vi "VMP_TestStand.vi"() -> ()   [LabVIEW 2016]
uses:
  <vilib>/userdefined/High Color/IMAQdx.ctl
  Enum_TypeDefinitions/Enum_TypeDef_FidMarkers.ctl
  Enum_TypeDefinitions/Enum_TypeDef_Sensors.ctl
  <vilib>/vision/Image Controls.llb/IMAQ Image.ctl
  <vilib>/Utility/file.llb/Read Delimited Spreadsheet (DBL).vi
  <vilib>/vision/driver/NI_Vision_Acquisition_Software.lvlib
panel:
  out "Module Progress Report":T1(array[cluster])
  in  "Reports path":path=path "C:/Users/Aerotech/cernbox/BNL/Stave Assembly Records/2017-05-10/ModulePlacement/5-11-2017"
  in  "Tab Control":enum32{"Camera", "Error handling"}(tab)
  in  "Camera Name":T2="cam1" caption="IMAQdx Session"
  in  "Camera gain":dbl
  in  "Module fiducial marker":T3
  in  "N modules":i32=2
  in  "Sensor Pattern":T4=enum."ATLAS12"
  out "Camera error out":errorcluster
  out "error out":errorcluster
  in  "Coordinates file path (dialog if empty)":path
  in  "Current module #":string
  in  "Current build phase":string
  in  "Axis Speeds":T5={"X [mm/s]"=25.0, "Y [mm/s]"=12.5, "Z [mm/s]"=5.0}
  in  "terminate":bool
  out "Current field of view":T6(plugin-control)
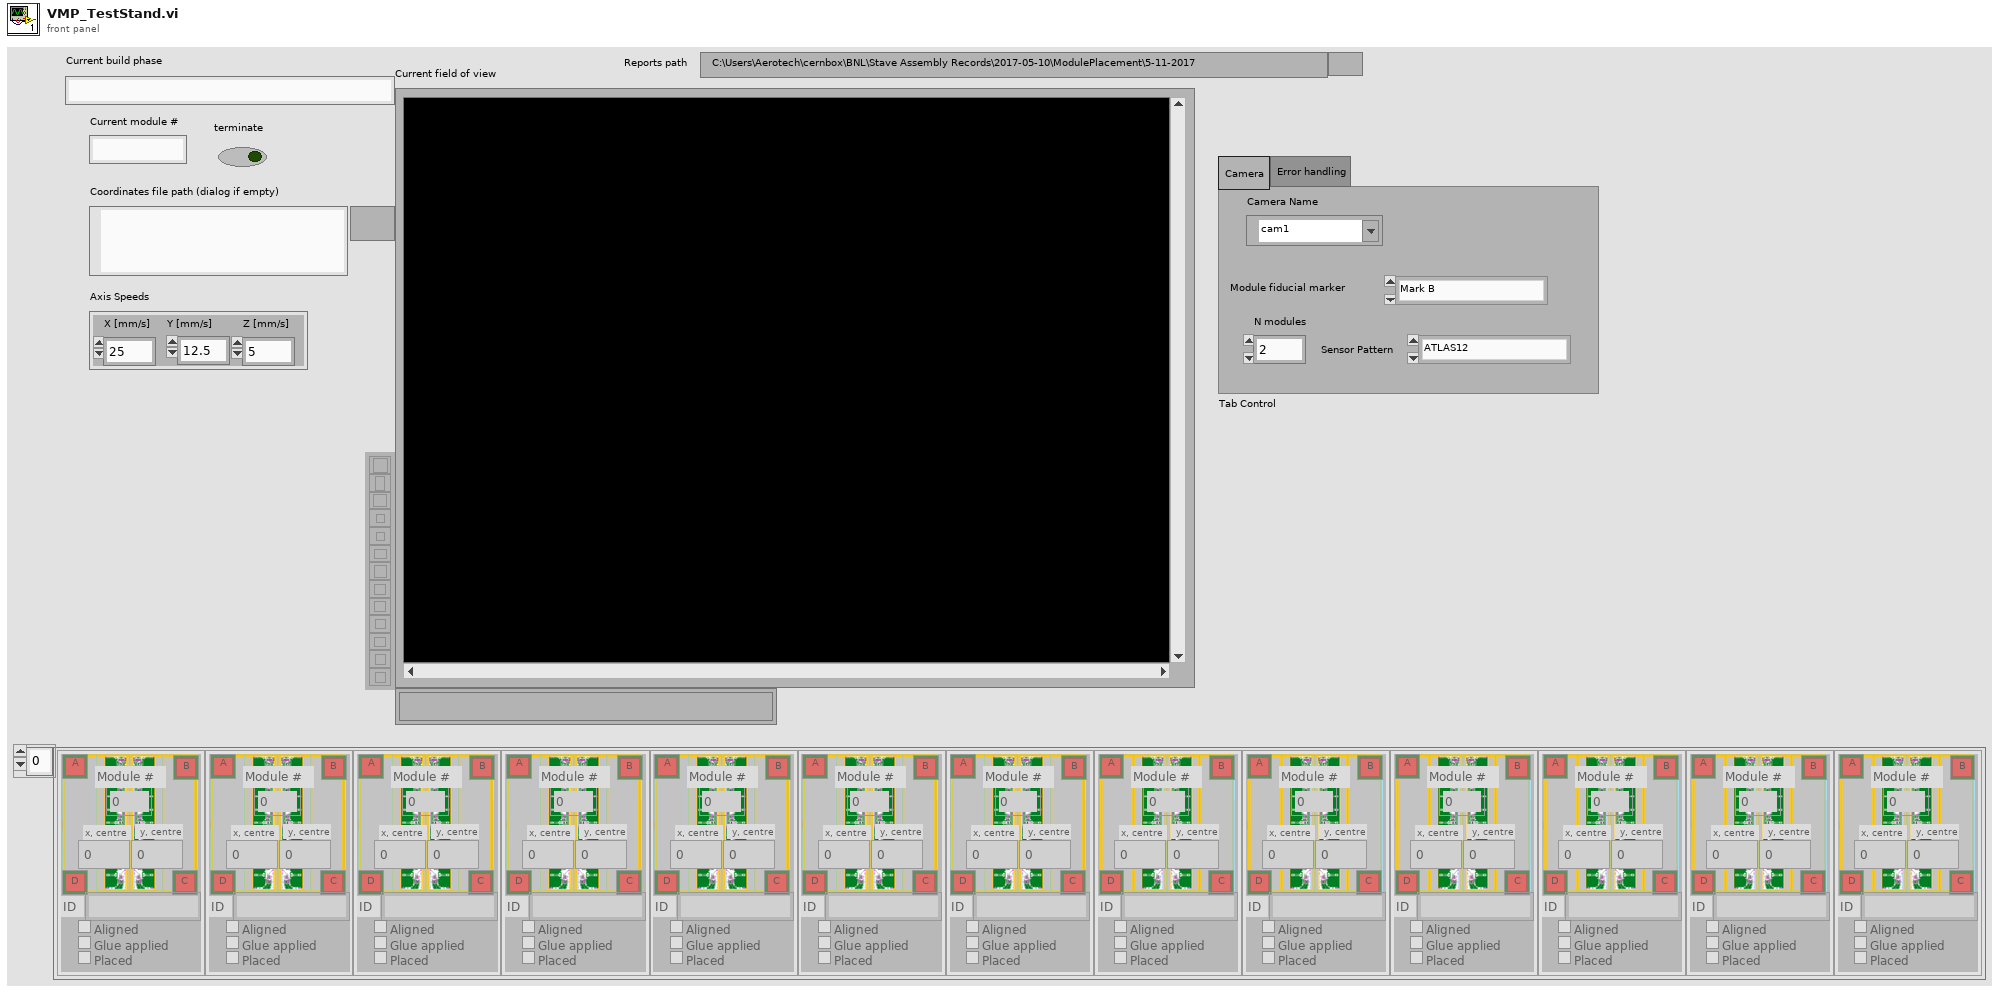
[diagram p1: front panel]
types:
  T1 = cluster{"B":bool, "A":bool, "D":bool, "C":bool, "ID":string, "Module #":i32, "x, centre":dbl, "y, centre":dbl, "Aligned":bool, "Glue applied":bool, "Placed":bool}[]
  T2 = typedef "IMAQdx.ctl" = refnum<k21>
  T3 = typedef "Enum_TypeDef_FidMarkers.ctl" = enum16{"Mark B", "Mark C", "Strip Corner", "Mark I (Slim/17)", "Mark E (Slim/17)", "Mark F (Slim/17)", "Mark G (Slim/17)", "Mark A (12)", "KaptonSpacers"}
  T4 = typedef "Enum_TypeDef_Sensors.ctl" = enum16{"ATLAS07", "ATLAS12", "ATLAS12Slim", "ATLAS17LS"}
  T5 = cluster{"X [mm/s]":dbl, "Y [mm/s]":dbl, "Z [mm/s]":dbl}
  T6 = typedef "IMAQ Image.ctl" = refnum<image>
  T7 = typedef "Image Type" = u32
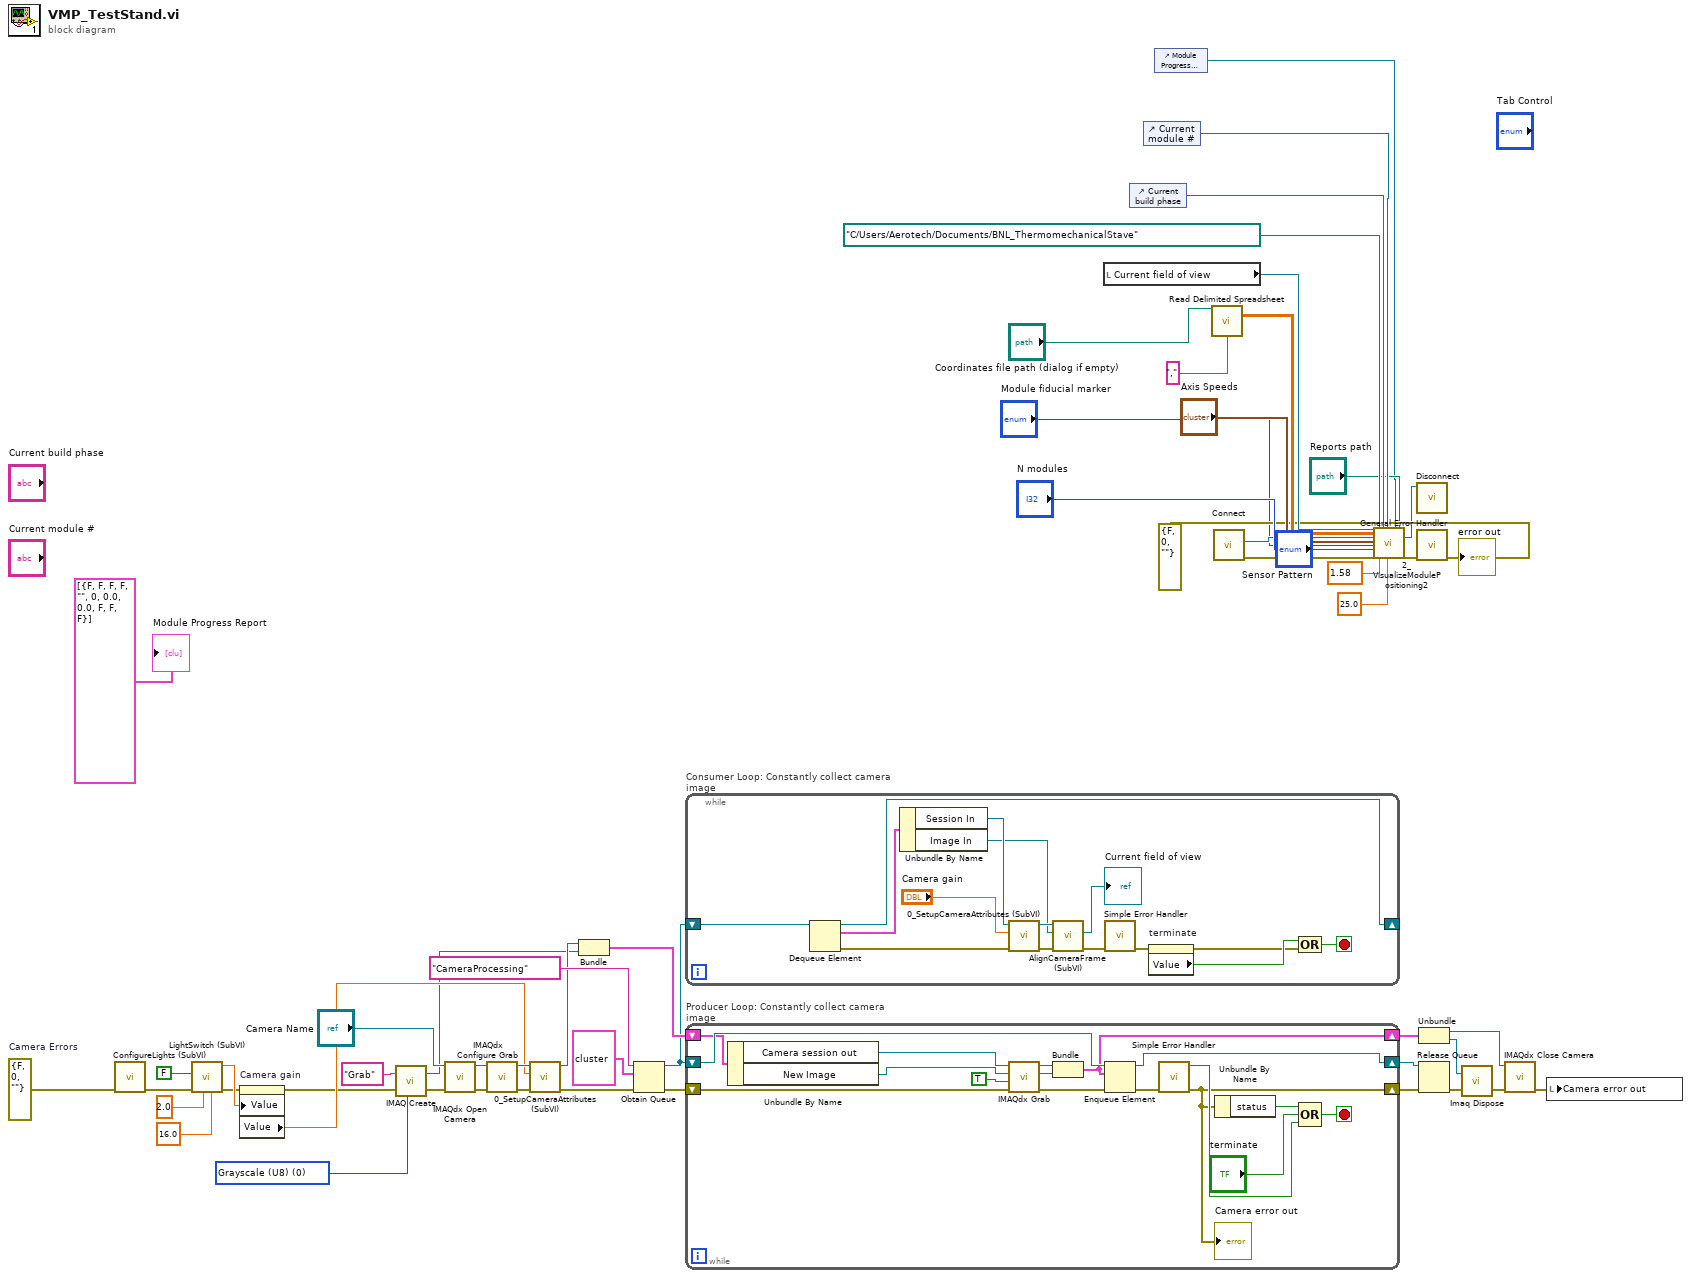
[diagram p0: block diagram]
diagram:
  w25 = errorcluster {"status"=FALSE, "code"=0, "source"=""}  # Camera Errors
  w53 = T7 0 items=["Grayscale (U8)", "Grayscale (I16)", "Grayscale (SGL)", "Complex (CSG)", "RGB (U32)", "HSL (U32)", "RGB (U64)", "Grayscale (U16)"] ("Image Type")
  n1 = call "ConfigureLights (SubVI).vi"("error in"=w25) -> ("error out"=w24:errorcluster)  [unwired: 10 in]
  n2 = call "LightSwitch (SubVI).vi"("Stave Gain"=16.0, "Si Gain"=2.0, "error in"=w24, "Spotlight"=FALSE) -> ("error out"=w45:errorcluster, "Assigned camera gain"=w46:dbl)  [unwired: 5 in, 1 out]
  n3 = property on="Camera gain" class="DigNum (strict)"(error in=w45, "Value"=w46) -> (error out=w23:errorcluster, "Value"=w40:dbl)  [unwired: 1 in, 1 out]
  n4 = call "IMAQ Create"("Image Name"="Grab", "Image Type"=w53, "error in (no error)"=w23) -> ("New Image"=w36:T6, "error out"=w50:errorcluster)  [unwired: 1 in, 1 out]
  n5 = call <vilib>:"IMAQdx Open Camera.vi"("error in"=w50, "Session In"="Camera Name") -> ("error out"=w51:errorcluster, "Session Out"=w54:T2)  [unwired: 1 in, 7 out]
  n6 = call <vilib>:"IMAQdx Configure Grab.vi"("error in"=w51, "Session In"=w54) -> ("error out"=w41:errorcluster, "Session Out"=w42:T2)  [unwired: 8 out]
  n7 = call "0_SetupCameraAttributes (SubVI).vi"("error in (no error)"=w41, "Gain"=w40, "Camera session in"=w42) -> ("error out"=w39:errorcluster, "Camera session out"=w37:T2)  [unwired: 7 in]
  n8 = Bundle("Camera session out"=w37, "New Image"=w36) -> (w35:cluster{"Camera session out":T2, "New Image":T6})  [unwired: 1 in]
  n9 = Obtain Queue(name (unnamed)="CameraProcessing", element data type=cluster{"Session In":T2, "Image In":T6} {"Session In"="", "Image In"=refnum}, error in (no error)=w39) -> (queue out=w27:refnum<queue>, error out=w38:errorcluster)  [unwired: 2 in, 1 out]
  n10 = while "Consumer Loop: Constantly collect camera image" {
    shift-right: [w65] -> _
    shift-left: w27 -> [w70]
    stop <- w68 stop-if-true
    n11 = Dequeue Element(queue=w70) -> (queue out=w65:refnum<queue>, element=w69:cluster{"Session In":T2, "Image In":T6}, error out=w67:errorcluster)  [unwired: 2 in, 1 out]
    n12 = Unbundle By Name(w69) -> ("Session In"=w64:T2, "Image In"=w62:T6)
    n13 = call "0_SetupCameraAttributes (SubVI).vi"("error in (no error)"=w67, "Gain"="Camera gain", "Camera session in"=w64) -> ("error out"=w61:errorcluster, "Camera session out"=w63:T2)  [unwired: 7 in]
    n14 = call "AlignCameraFrame (SubVI).vi"("error in (no error)"=w61, "Image Src"=w62, "Camera session in"=w63) -> ("error out"=w59:errorcluster, "Image Dst Out"=→"Current field of view":T6)  [unwired: 6 in, 1 out]
    n15 = call <vilib>:"Simple Error Handler.vi"("error in (no error)"=w59) -> ("error out"=w58:errorcluster)  [unwired: 4 in, 4 out]
    n16 = property on="terminate" class="Bool (strict)"(error in=w58) -> (error out=w57:errorcluster, "Value"=w66:bool)  [unwired: 1 in, 1 out]
    n17 = Compound Arithmetic op=OR(w66, w57) -> (w68:bool)
  }
  n18 = while "Producer Loop: Constantly collect camera image" {
    shift-right: [w84] -> w34
    shift-left: w27 -> [w85]
    shift-right: [w73] -> w33
    shift-left: w38 -> [w86]
    shift-right: [w75] -> w32
    shift-left: w35 -> [w78]
    stop <- w74 stop-if-true
    n19 = Unbundle By Name(w78) -> ("Camera session out"=w77:T2, "New Image"=w76:T6)
    n20 = call <vilib>:"IMAQdx Grab.vi"("error in"=w86, "Wait for Next Buffer? (Yes)"=TRUE, "Image In"=w76, "Session In"=w77) -> ("error out"=w83:errorcluster, "Image Out"=w79:T6, "Session Out"=w80:T2)  [unwired: 5 out]
    n21 = Bundle("Session Out"=w80, "Image Out"=w79) -> (w75:cluster{"Session Out":T2, "Image Out":T6})  [unwired: 1 in]
    n22 = Enqueue Element(queue=w85, element=w75, error in (no error)=w83) -> (queue out=w84:refnum<queue>, error out=w82:errorcluster)  [unwired: 1 in, 1 out]
    n23 = call <vilib>:"Simple Error Handler.vi"("error in (no error)"=w82) -> ("error?"=w87:bool, "error out"=w73:errorcluster)  [unwired: 4 in, 3 out]
    "Camera error out" <- w73
    n24 = Unbundle By Name(w73) -> ("status"=w81:bool)
    n25 = Compound Arithmetic op=OR(w81, "terminate", w87) -> (w74:bool)
  }
  n26 = local read "Current field of view"() -> (w16:T6)
  n27 = control-ref of="Current build phase"() -> (w11:refnum<vi>)
  n28 = control-ref of="Current module #"() -> (w12:refnum<vi>)
  n29 = control-ref of="Module Progress Report"() -> (w1:refnum<vi>)
  n30 = call-poly <vilib>:"Read Delimited Spreadsheet.vi"("file path (dialog if empty)"="Coordinates file path (dialog if empty)", "delimiter (\\t)"="," ("delimiter (\\t)")) -> ("all rows"=w14:dbl[][])  [unwired: 8 in, 5 out]
  n31 = call "Connect.vi"("error in (no error)"=errorcluster {"status"=FALSE, "code"=0, "source"=""} ("error in")) -> ("error out"=w7:errorcluster, "controller"=w10:refnum<k24>)  [unwired: 9 in]
  n32 = call "2_VisualizeModulePositioning2.vi"("Placement Monitor"=w16, "Calibrated positions of fiducials [mm]"=w14, "XYZ .NET Refnum in"=w10, "Axis Speeds"="Axis Speeds", "Module fiducial marker"="Module fiducial marker", "N modules"="N modules", "Sensor Pattern"="Sensor Pattern", "error in (no error)"=w7, "Templates path"=path "C:/Users/Aerotech/Documents/BNL_ThermomechanicalStave", "Calibration [um/pix]"=1.58, "Current Build Phase"=w11, "Module #"=w12, "Placement tolerance [um]"=25.0, "Module Report"=w1, "Reports path"="Reports path") -> ("XYZ .NET Refnum out"=w8:refnum<k24>, "error out"=w21:errorcluster)  [unwired: 11 in]
  n33 = call "Disconnect.vi"("controller"=w8) -> ()  [unwired: 10 in, 1 out]
  n34 = call <vilib>:"General Error Handler.vi"("error in (no error)"=w21) -> ("error out"=→"error out":errorcluster)  [unwired: 10 in, 4 out]
  n35 = Unbundle(w32) -> ("Camera session out"=w31:T2, "New Image"=w30:T6)
  n36 = Release Queue(queue=w34, error in (no error)=w33) -> (error out=w28:errorcluster)  [unwired: 1 in, 2 out]
  n37 = call "Imaq Dispose"("Image"=w30, "error in (no error)"=w28) -> ("error out"=w29:errorcluster)  [unwired: 4 in]
  n38 = call <vilib>:"IMAQdx Close Camera.vi"("error in"=w29, "Session In"=w31) -> ("error out"=w26:errorcluster)  [unwired: 9 in]
  n39 = local write "Camera error out"(w26) -> ()
  "Module Progress Report" <- T1 [{"B"=FALSE, "A"=FALSE, "D"=FALSE, "C"=FALSE, "ID"="", "Module #"=0, "x, centre"=0.0, "y, centre"=0.0, "Aligned"=FALSE, "Glue applied"=FALSE, "Placed"=FALSE}] ("Module Progress Report")
